vi "Test Move Columns.vi"(8 "error in (no error)":errorcluster) -> (0 "error out":errorcluster)   [LabVIEW 2019, in "LV-Data.PGSQL.lvclass"]
uses:
  LV-Data.PGSQL.lvclass
panel:
  out "LV-Data.PG out":refnum<class "LV-Data.PGSQL.lvclass">
  in  "LV-Data.PG in":refnum<class "LV-Data.PGSQL.lvclass">
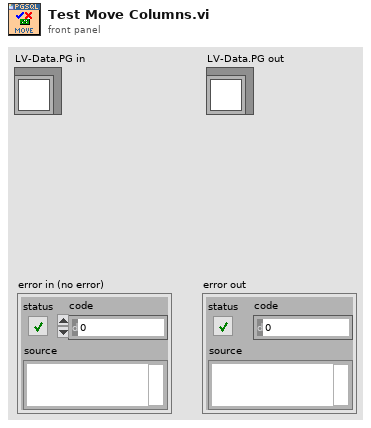
[diagram p1: front panel]
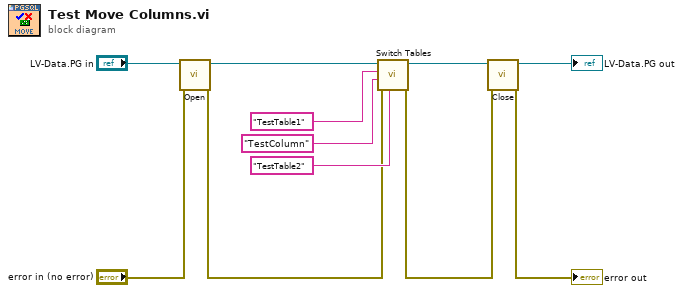
[diagram p0: block diagram]
diagram:
  n1 = call-dynamic "Open.vi"("error in (no error)"="error in (no error)", "Data.PG in"="LV-Data.PG in") -> ("error out"=w2:errorcluster, "Data.PG out"=w4:refnum<class "LV-Data.PGSQL.lvclass">)  [unwired: 8 in]
  n2 = call "Switch Tables.vi"("New Table Name"="TestTable2" ("New Table"), "error in (no error)"=w2, "Column Name"="TestColumn" ("Old Column"), "Old Table Name"="TestTable1" ("Old Table"), "Data.PG"=w4) -> ("error out"=w1:errorcluster, "Data.PG out"=w3:refnum<class "LV-Data.PGSQL.lvclass">)  [unwired: 5 in]
  n3 = call-dynamic "Close.vi"("error in (no error)"=w1, "Data.PG in"=w3) -> ("error out"=→"error out":errorcluster, "Data.PG out"=→"LV-Data.PG out":refnum<class "LV-Data.PGSQL.lvclass">)  [unwired: 8 in]
